vi "Power Qualtiy - 5.vi"() -> ()   [LabVIEW 2015]
uses:
  <vilib>/measure/matone.llb/Harmonic Distortion Analyzer N Chan.vi
  <vilib>/express/express analysis/Spectral/Block/exnSpectralBlock spectral measurements RMS poly.vi
  <vilib>/express/express analysis/Spectral/Block/exnSpectralBlock spectral measurements RMS DDT.vi
  <vilib>/express/express analysis/Spectral/XNode/ExpressSpectralMeasurementsBlockNode.xnode
  <vilib>/measure/NI_MAPro.lvlib
panel:
  in  "file":path
  out "components levels":cluster{"components level":dbl[]}[](array[cluster]) {"components level" format="%.2p"}
  out "detected fundamental frequencies":dbl[](array[numeric]) format="%.2p"
  out "Voltage Waveform":dynamicdata(graph)
  out "Current Waveform":dynamicdata(graph)
  out "Current":dbl(knob) scale=0.0..12.0
  out "Voltage":dbl(knob) scale=0.0..230.0
  out "THD":dbl
  out "Current Harmonics":dynamicdata(graph)
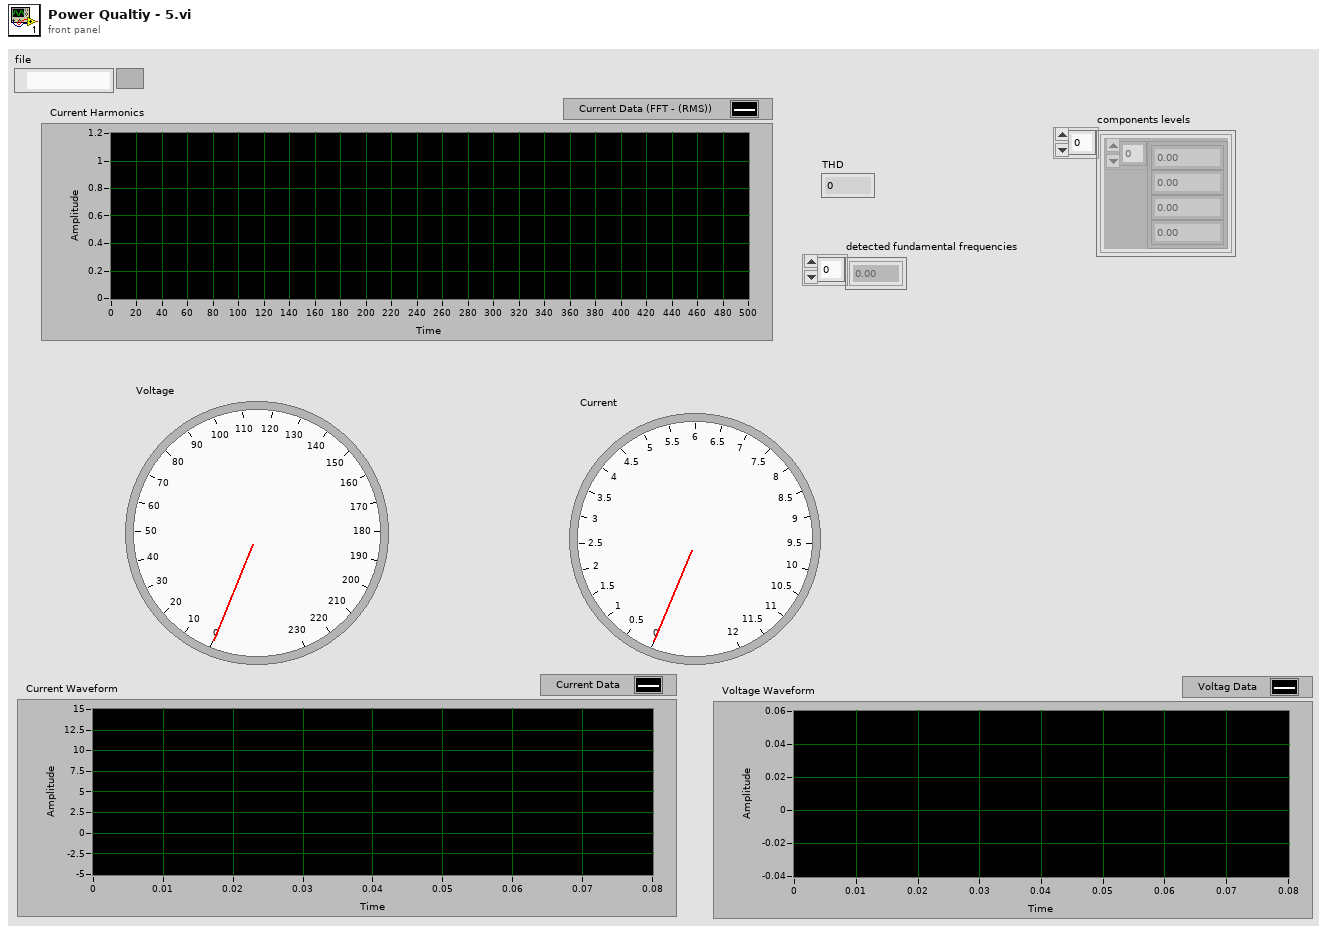
[diagram p1: front panel]
types:
  T1 = enum16{"open", "open or create", "create or replace", "create", "open (read-only)"}
  T2 = enum16{"none", "input signal", "fundamental signal", "residual signal", "harmonics only", "noise and spurs"}
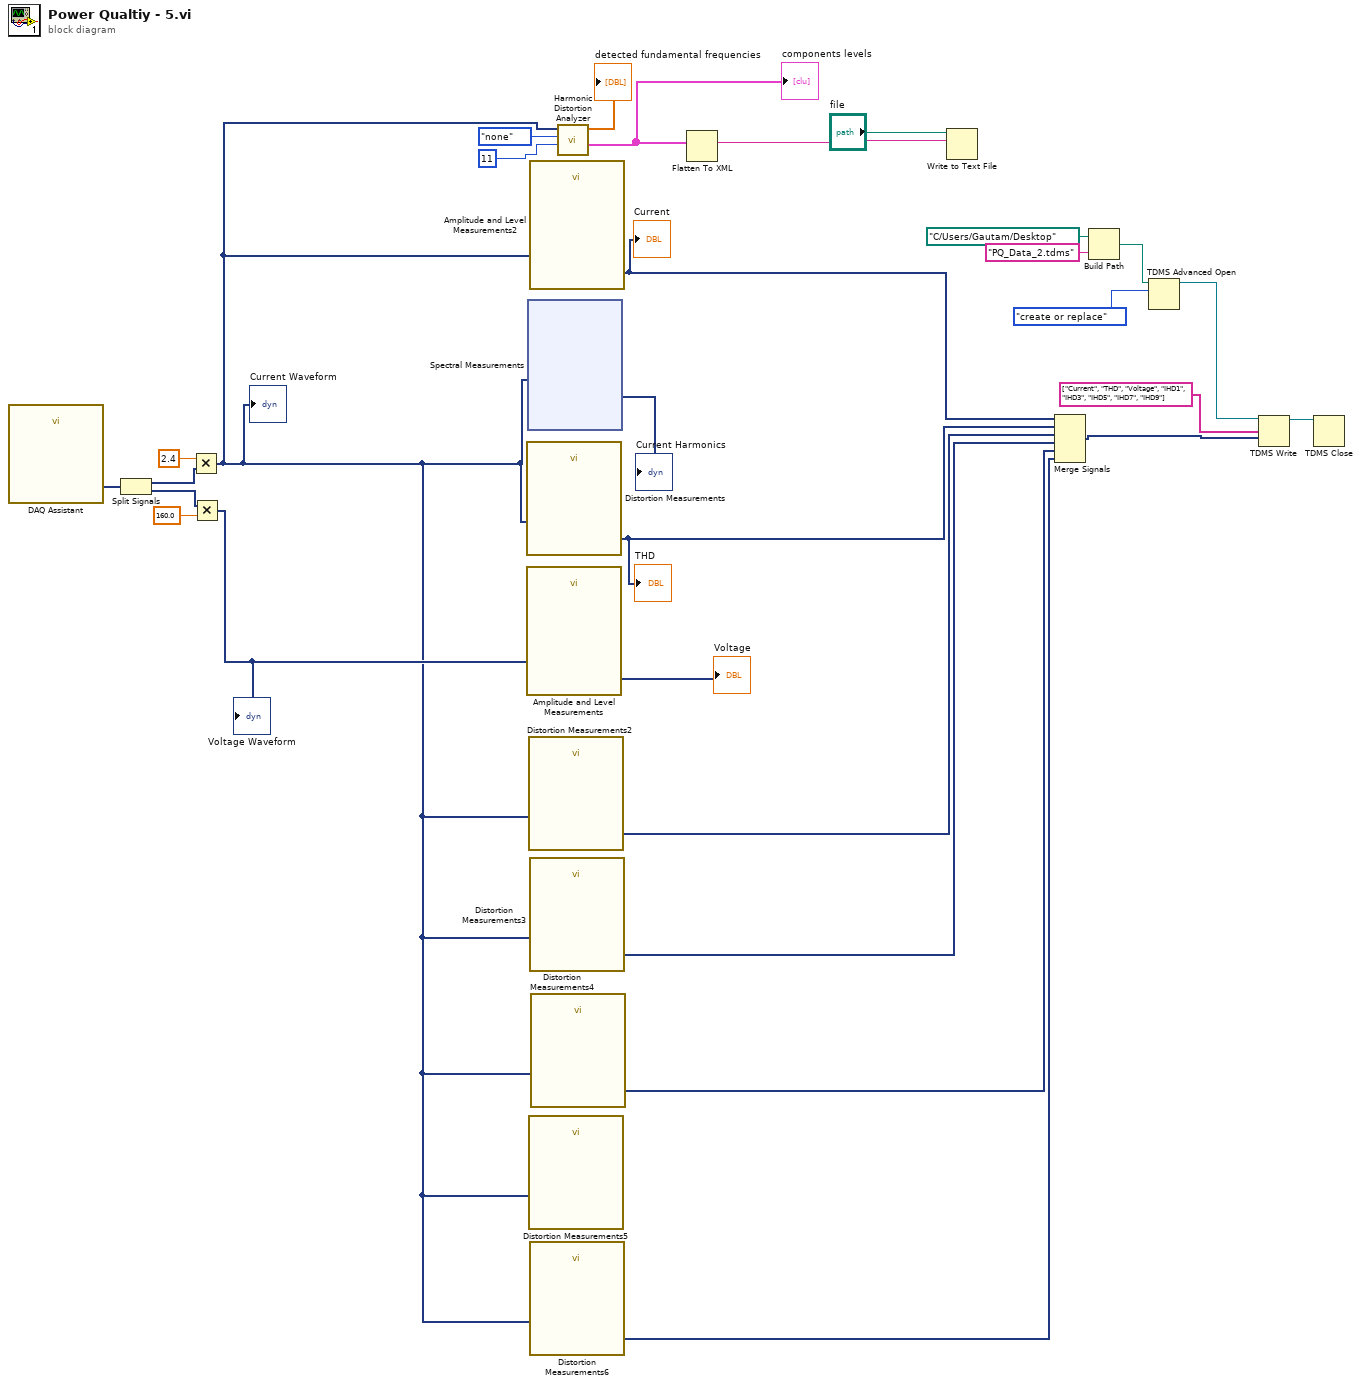
[diagram p0: block diagram]
diagram:
  n1 = call "DAQ Assistant"() -> ("data"=w29:dynamicdata)  [unwired: 17 in, 2 out]
  n2 = Split Signals(w29) -> (w28:dynamicdata, w27:dynamicdata)  [unwired: 2 in]
  n3 = Multiply(x=2.4, y=w28) -> (x*y=w16:dynamicdata)
  "Current Waveform" <- w16
  n4 = Multiply(x=w27, y=160.0) -> (x*y=w24:dynamicdata)
  "Voltage Waveform" <- w24
  n5 = call "Distortion Measurements"("Signals"=w16) -> ("THD"=w14:dynamicdata)  [unwired: 9 in, 1 out]
  "THD" <- w14
  n6 = call "Amplitude and Level Measurements"("Signals"=w24) -> ("RMS"=→"Voltage":dynamicdata)  [unwired: 13 in, 1 out]
  n7 = xnode "Spectral Measurements"("Signals"=w16) -> ("FFT - (RMS)"=→"Current Harmonics":dynamicdata)  [unwired: 1 in, 2 out]
  n8 = call "Distortion Measurements2"("Signals"=w16) -> ("Specific Harmonic"=w13:dynamicdata)  [unwired: 9 in, 1 out]
  n9 = call "Distortion Measurements5"("Signals"=w16) -> ()  [unwired: 9 in, 2 out]
  n10 = call "Amplitude and Level Measurements2"("Signals"=w16) -> ("RMS"=w10:dynamicdata)  [unwired: 13 in, 1 out]
  "Current" <- w10
  n11 = call "Distortion Measurements3"("Signals"=w16) -> ("Specific Harmonic"=w12:dynamicdata)  [unwired: 9 in, 1 out]
  n12 = call "Distortion Measurements6"("Signals"=w16) -> ("Specific Harmonic"=w9:dynamicdata)  [unwired: 9 in, 1 out]
  n13 = call "Distortion Measurements4"("Signals"=w16) -> ("Specific Harmonic"=w11:dynamicdata)  [unwired: 9 in, 1 out]
  n14 = call-poly <vilib>:"Harmonic Distortion Analyzer.vi"("highest harmonic"=11, "export mode"=T2."none", "signals in"=w16) -> ("components levels"=w17:cluster{"components level":dbl[]}[], "detected fundamental frequencies"=→"detected fundamental frequencies":dbl[])  [unwired: 3 in, 4 out]
  "components levels" <- w17
  n15 = Flatten To XML(anything=w17) -> (xml string=w19:string)
  n16 = Write to Text File(file (use dialog)="file", text=w19) -> ()  [unwired: 2 in, 3 out]
  n17 = Merge Signals(w10, w14, w13, w12, w11, w9) -> (w1:dynamicdata)
  n18 = Build Path(base path=path "C:/Users/Gautam/Desktop", name or relative path="PQ_Data_2.tdms") -> (appended path=w7:path)
  n19 = TDMS Advanced Open(10:T1."create or replace" ("operation (0:open)"), 11:w7) -> (3:w3:refnum<k34>)  [unwired: 3 in, 2 out]
  n20 = TDMS Write(0:w3, 7:string[] ["Current", "THD", "Voltage", "IHD1", "IHD3", "IHD5", "IHD7", "IHD9"] ("channel name(s) in (Untitled)"), 9:w1) -> (4:w4:refnum<k34>)  [unwired: 3 in, 3 out]
  n21 = TDMS Close(11:w4) -> ()  [unwired: 1 in, 2 out]
